vi "readTelemetryFPGAData.vi"(8 "error in (no error)":errorcluster, 10 "Parser":refnum<class "U8ArrayParserAutoIndexing.lvclass">, 11 "M1M3SAL in":refnum<class "M1M3SAL.lvclass">) -> (0 "error out":errorcluster, 2 "EventSummaryState":variant, 3 "M1M3SAL out":refnum<class "M1M3SAL.lvclass">)   [LabVIEW 2016, in "M1M3SupportCommunicator.lvlib" / "M1M3SAL.lvclass"]
uses:
  M1M3SAL.lvclass
  Common_RT_Utilities/U8ArrayParserAutoIndexing/U8ArrayParserAutoIndexing.lvclass
  DataTypes/Topics/TelemetryFPGAData.ctl
  DataTypes/Topics/Parts/Timestamp.ctl
  DataTypes/Topics/M1M3SupportTopics.lvlib
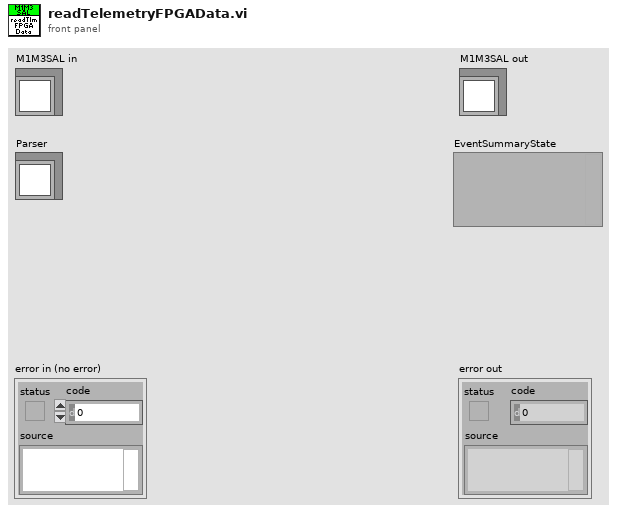
[diagram p1: front panel]
types:
  T1 = typedef "M1M3SupportTopics.lvlib/TelemetryFPGAData.ctl" = cluster{"Timestamp":T2, "ModbusSubnetATxInternalFIFOOverflow":bool, "ModbusSubnetAInvalidInstruction":bool, "ModbusSubnetAWaitForRxFrameTimeout":bool, "ModbusSubnetAStartBitError":bool, "ModbusSubnetAStopBitError":bool, "ModbusSubnetARxDataFIFOOverflow":bool, "ModbusSubnetATxByteCount":u32, "ModbusSubnetATxFrameCount":u32, "ModbusSubnetARxByteCount":u32, "ModbusSubnetARxFrameCount":u32, "ModbusSubnetBTxInternalFIFOOverflow":bool, "ModbusSubnetBInvalidInstruction":bool, "ModbusSubnetBWaitForRxFrameTimeout":bool, "ModbusSubnetBStartBitError":bool, "ModbusSubnetBStopBitError":bool, "ModbusSubnetBRxDataFIFOOverflow":bool, "ModbusSubnetBTxByteCount":u32, "ModbusSubnetBTxFrameCount":u32, "ModbusSubnetBRxByteCount":u32, "ModbusSubnetBRxFrameCount":u32, "ModbusSubnetCTxInternalFIFOOverflow":bool, "ModbusSubnetCInvalidInstruction":bool, "ModbusSubnetCWaitForRxFrameTimeout":bool, "ModbusSubnetCStartBitError":bool, "ModbusSubnetCStopBitError":bool, "ModbusSubnetCRxDataFIFOOverflow":bool, "ModbusSubnetCTxByteCount":u32, "ModbusSubnetCTxFrameCount":u32, "ModbusSubnetCRxByteCount":u32, "ModbusSubnetCRxFrameCount":u32, "ModbusSubnetDTxInternalFIFOOverflow":bool, "ModbusSubnetDInvalidInstruction":bool, "ModbusSubnetDWaitForRxFrameTimeout":bool, "ModbusSubnetDStartBitError":bool, "ModbusSubnetDStopBitError":bool, "ModbusSubnetDRxDataFIFOOverflow":bool, "ModbusSubnetDTxByteCount":u32, "ModbusSubnetDTxFrameCount":u32, "ModbusSubnetDRxByteCount":u32, "ModbusSubnetDRxFrameCount":u32, "ModbusSubnetETxInternalFIFOOverflow":bool, "ModbusSubnetEInvalidInstruction":bool, "ModbusSubnetEWaitForRxFrameTimeout":bool, "ModbusSubnetEStartBitError":bool, "ModbusSubnetEStopBitError":bool, "ModbusSubnetERxDataFIFOOverflow":bool, "ModbusSubnetETxByteCount":u32, "ModbusSubnetETxFrameCount":u32, "ModbusSubnetERxByteCount":u32, "ModbusSubnetERxFrameCount":u32, "FPGATimestamp":dbl}
  T2 = typedef "M1M3SupportTopics.lvlib/Timestamp.ctl" = dbl
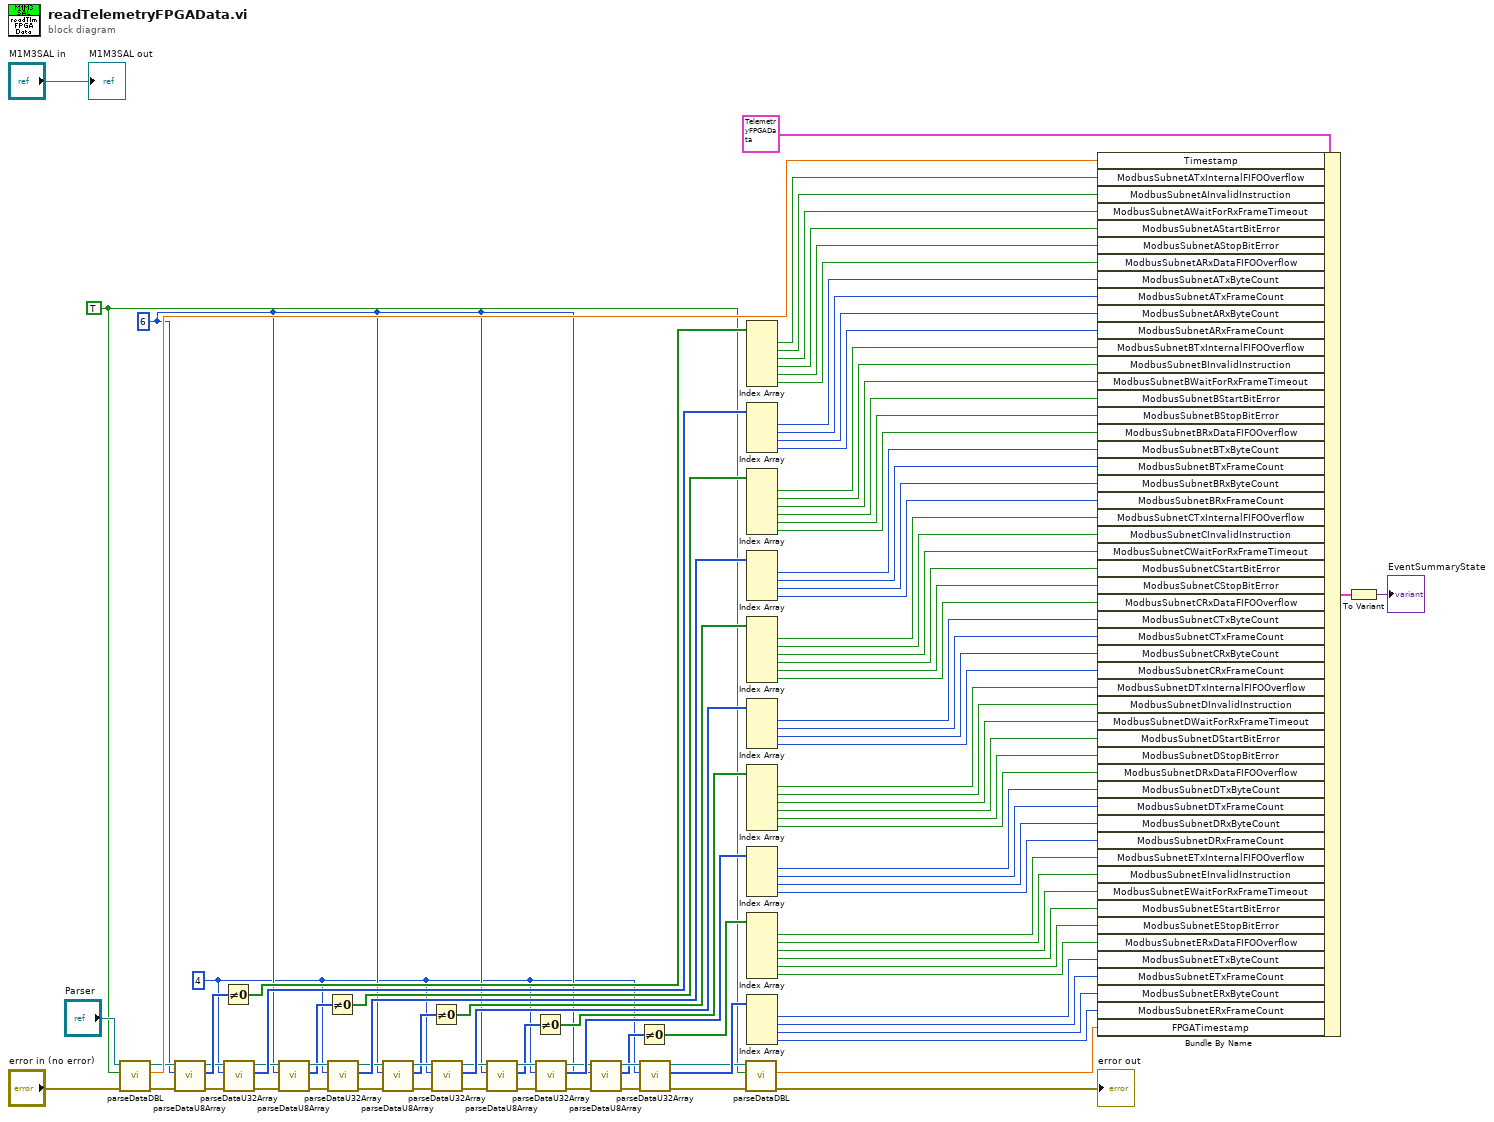
[diagram p0: block diagram]
diagram:
  w1 = TRUE ("OverrideSwapBytes")
  w2 = 4 ("Length")
  w3 = 6 ("Length")
  n1 = call "parseDataDBL.vi"("error in (no error)"="error in (no error)", "OverrideSwapBytes"=w1, "U8ArrayParserAutoIndexing in"="Parser") -> ("error out"=w76:errorcluster, "Data"=w94:dbl, "U8ArrayParserAutoIndexing out"=w79:refnum<class "U8ArrayParserAutoIndexing.lvclass">)  [unwired: 6 in]
  n2 = call "parseDataU8Array.vi"("U8ArrayParserAutoIndexing in"=w79, "Length"=w3, "error in (no error)"=w76) -> ("U8ArrayParserAutoIndexing out"=w78:refnum<class "U8ArrayParserAutoIndexing.lvclass">, "Data"=w92:u8[], "error out"=w75:errorcluster)  [unwired: 5 in]
  n3 = Not Equal To 0?(x=w92) -> (x != 0?=w91:bool[])
  n4 = call "parseDataU32Array.vi"("U8ArrayParserAutoIndexing in"=w78, "Length"=w2, "error in (no error)"=w75) -> ("U8ArrayParserAutoIndexing out"=w77:refnum<class "U8ArrayParserAutoIndexing.lvclass">, "Data"=w83:u32[], "error out"=w74:errorcluster)  [unwired: 5 in]
  n5 = call "parseDataU8Array.vi"("U8ArrayParserAutoIndexing in"=w77, "Length"=w3, "error in (no error)"=w74) -> ("U8ArrayParserAutoIndexing out"=w73:refnum<class "U8ArrayParserAutoIndexing.lvclass">, "Data"=w72:u8[], "error out"=w12:errorcluster)  [unwired: 5 in]
  n6 = Not Equal To 0?(x=w72) -> (x != 0?=w71:bool[])
  n7 = call "parseDataU32Array.vi"("U8ArrayParserAutoIndexing in"=w73, "Length"=w2, "error in (no error)"=w12) -> ("U8ArrayParserAutoIndexing out"=w69:refnum<class "U8ArrayParserAutoIndexing.lvclass">, "Data"=w70:u32[], "error out"=w11:errorcluster)  [unwired: 5 in]
  n8 = call "parseDataU8Array.vi"("U8ArrayParserAutoIndexing in"=w69, "Length"=w3, "error in (no error)"=w11) -> ("U8ArrayParserAutoIndexing out"=w68:refnum<class "U8ArrayParserAutoIndexing.lvclass">, "Data"=w67:u8[], "error out"=w10:errorcluster)  [unwired: 5 in]
  n9 = Not Equal To 0?(x=w67) -> (x != 0?=w66:bool[])
  n10 = call "parseDataU32Array.vi"("U8ArrayParserAutoIndexing in"=w68, "Length"=w2, "error in (no error)"=w10) -> ("U8ArrayParserAutoIndexing out"=w64:refnum<class "U8ArrayParserAutoIndexing.lvclass">, "Data"=w65:u32[], "error out"=w9:errorcluster)  [unwired: 5 in]
  n11 = call "parseDataU8Array.vi"("U8ArrayParserAutoIndexing in"=w64, "Length"=w3, "error in (no error)"=w9) -> ("U8ArrayParserAutoIndexing out"=w63:refnum<class "U8ArrayParserAutoIndexing.lvclass">, "Data"=w62:u8[], "error out"=w8:errorcluster)  [unwired: 5 in]
  n12 = Not Equal To 0?(x=w62) -> (x != 0?=w61:bool[])
  n13 = call "parseDataU32Array.vi"("U8ArrayParserAutoIndexing in"=w63, "Length"=w2, "error in (no error)"=w8) -> ("U8ArrayParserAutoIndexing out"=w59:refnum<class "U8ArrayParserAutoIndexing.lvclass">, "Data"=w60:u32[], "error out"=w7:errorcluster)  [unwired: 5 in]
  n14 = call "parseDataU8Array.vi"("U8ArrayParserAutoIndexing in"=w59, "Length"=w3, "error in (no error)"=w7) -> ("U8ArrayParserAutoIndexing out"=w58:refnum<class "U8ArrayParserAutoIndexing.lvclass">, "Data"=w57:u8[], "error out"=w6:errorcluster)  [unwired: 5 in]
  n15 = Not Equal To 0?(x=w57) -> (x != 0?=w56:bool[])
  n16 = call "parseDataU32Array.vi"("U8ArrayParserAutoIndexing in"=w58, "Length"=w2, "error in (no error)"=w6) -> ("U8ArrayParserAutoIndexing out"=w54:refnum<class "U8ArrayParserAutoIndexing.lvclass">, "Data"=w55:u32[], "error out"=w5:errorcluster)  [unwired: 5 in]
  n17 = call "parseDataDBL.vi"("error in (no error)"=w5, "OverrideSwapBytes"=w1, "U8ArrayParserAutoIndexing in"=w54) -> ("error out"=→"error out":errorcluster, "Data"=w53:dbl)  [unwired: 6 in, 1 out]
  n18 = Index Array(array=w91) -> (element #1=w90:bool, element #2=w89:bool, element #3=w88:bool, element #4=w87:bool, element #5=w86:bool, element #6=w85:bool)  [unwired: 6 in]
  n19 = Index Array(array=w83) -> (element #1=w84:u32, element #2=w82:u32, element #3=w81:u32, element #4=w80:u32)  [unwired: 4 in]
  n20 = Index Array(array=w71) -> (element #1=w52:bool, element #2=w51:bool, element #3=w50:bool, element #4=w49:bool, element #5=w48:bool, element #6=w47:bool)  [unwired: 6 in]
  n21 = Index Array(array=w70) -> (element #1=w46:u32, element #2=w45:u32, element #3=w44:u32, element #4=w43:u32)  [unwired: 4 in]
  n22 = Index Array(array=w66) -> (element #1=w42:bool, element #2=w41:bool, element #3=w40:bool, element #4=w39:bool, element #5=w38:bool, element #6=w37:bool)  [unwired: 6 in]
  n23 = Index Array(array=w65) -> (element #1=w36:u32, element #2=w35:u32, element #3=w34:u32, element #4=w33:u32)  [unwired: 4 in]
  n24 = Index Array(array=w61) -> (element #1=w32:bool, element #2=w31:bool, element #3=w30:bool, element #4=w29:bool, element #5=w28:bool, element #6=w27:bool)  [unwired: 6 in]
  n25 = Index Array(array=w60) -> (element #1=w26:u32, element #2=w25:u32, element #3=w24:u32, element #4=w23:u32)  [unwired: 4 in]
  n26 = Index Array(array=w56) -> (element #1=w22:bool, element #2=w21:bool, element #3=w20:bool, element #4=w19:bool, element #5=w18:bool, element #6=w17:bool)  [unwired: 6 in]
  n27 = Index Array(array=w55) -> (element #1=w16:u32, element #2=w15:u32, element #3=w14:u32, element #4=w13:u32)  [unwired: 4 in]
  n28 = Bundle By Name(cluster=T1 {"Timestamp"=0.0, "ModbusSubnetATxInternalFIFOOverflow"=FALSE, "ModbusSubnetAInvalidInstruction"=FALSE, "ModbusSubnetAWaitForRxFrameTimeout"=FALSE, "ModbusSubnetAStartBitError"=FALSE, "ModbusSubnetAStopBitError"=FALSE, "ModbusSubnetARxDataFIFOOverflow"=FALSE, "ModbusSubnetATxByteCount"=0, "ModbusSubnetATxFrameCount"=0, "ModbusSubnetARxByteCount"=0, "ModbusSubnetARxFrameCount"=0, "ModbusSubnetBTxInternalFIFOOverflow"=FALSE, "ModbusSubnetBInvalidInstruction"=FALSE, "ModbusSubnetBWaitForRxFrameTimeout"=FALSE, "ModbusSubnetBStartBitError"=FALSE, "ModbusSubnetBStopBitError"=FALSE, "ModbusSubnetBRxDataFIFOOverflow"=FALSE, "ModbusSubnetBTxByteCount"=0, "ModbusSubnetBTxFrameCount"=0, "ModbusSubnetBRxByteCount"=0, "ModbusSubnetBRxFrameCount"=0, "ModbusSubnetCTxInternalFIFOOverflow"=FALSE, "ModbusSubnetCInvalidInstruction"=FALSE, "ModbusSubnetCWaitForRxFrameTimeout"=FALSE, "ModbusSubnetCStartBitError"=FALSE, "ModbusSubnetCStopBitError"=FALSE, "ModbusSubnetCRxDataFIFOOverflow"=FALSE, "ModbusSubnetCTxByteCount"=0, "ModbusSubnetCTxFrameCount"=0, "ModbusSubnetCRxByteCount"=0, "ModbusSubnetCRxFrameCount"=0, "ModbusSubnetDTxInternalFIFOOverflow"=FALSE, "ModbusSubnetDInvalidInstruction"=FALSE, "ModbusSubnetDWaitForRxFrameTimeout"=FALSE, "ModbusSubnetDStartBitError"=FALSE, "ModbusSubnetDStopBitError"=FALSE, "ModbusSubnetDRxDataFIFOOverflow"=FALSE, "ModbusSubnetDTxByteCount"=0, "ModbusSubnetDTxFrameCount"=0, "ModbusSubnetDRxByteCount"=0, "ModbusSubnetDRxFrameCount"=0, "ModbusSubnetETxInternalFIFOOverflow"=FALSE, "ModbusSubnetEInvalidInstruction"=FALSE, "ModbusSubnetEWaitForRxFrameTimeout"=FALSE, "ModbusSubnetEStartBitError"=FALSE, "ModbusSubnetEStopBitError"=FALSE, "ModbusSubnetERxDataFIFOOverflow"=FALSE, "ModbusSubnetETxByteCount"=0, "ModbusSubnetETxFrameCount"=0, "ModbusSubnetERxByteCount"=0, "ModbusSubnetERxFrameCount"=0, "FPGATimestamp"=0.0} ("TelemetryFPGAData"), "Timestamp"=w94, "ModbusSubnetATxInternalFIFOOverflow"=w90, "ModbusSubnetAInvalidInstruction"=w89, "ModbusSubnetAWaitForRxFrameTimeout"=w88, "ModbusSubnetAStartBitError"=w87, "ModbusSubnetAStopBitError"=w86, "ModbusSubnetARxDataFIFOOverflow"=w85, "ModbusSubnetATxByteCount"=w84, "ModbusSubnetATxFrameCount"=w82, "ModbusSubnetARxByteCount"=w81, "ModbusSubnetARxFrameCount"=w80, "ModbusSubnetBTxInternalFIFOOverflow"=w52, "ModbusSubnetBInvalidInstruction"=w51, "ModbusSubnetBWaitForRxFrameTimeout"=w50, "ModbusSubnetBStartBitError"=w49, "ModbusSubnetBStopBitError"=w48, "ModbusSubnetBRxDataFIFOOverflow"=w47, "ModbusSubnetBTxByteCount"=w46, "ModbusSubnetBTxFrameCount"=w45, "ModbusSubnetBRxByteCount"=w44, "ModbusSubnetBRxFrameCount"=w43, "ModbusSubnetCTxInternalFIFOOverflow"=w42, "ModbusSubnetCInvalidInstruction"=w41, "ModbusSubnetCWaitForRxFrameTimeout"=w40, "ModbusSubnetCStartBitError"=w39, "ModbusSubnetCStopBitError"=w38, "ModbusSubnetCRxDataFIFOOverflow"=w37, "ModbusSubnetCTxByteCount"=w36, "ModbusSubnetCTxFrameCount"=w35, "ModbusSubnetCRxByteCount"=w34, "ModbusSubnetCRxFrameCount"=w33, "ModbusSubnetDTxInternalFIFOOverflow"=w32, "ModbusSubnetDInvalidInstruction"=w31, "ModbusSubnetDWaitForRxFrameTimeout"=w30, "ModbusSubnetDStartBitError"=w29, "ModbusSubnetDStopBitError"=w28, "ModbusSubnetDRxDataFIFOOverflow"=w27, "ModbusSubnetDTxByteCount"=w26, "ModbusSubnetDTxFrameCount"=w25, "ModbusSubnetDRxByteCount"=w24, "ModbusSubnetDRxFrameCount"=w23, "ModbusSubnetETxInternalFIFOOverflow"=w22, "ModbusSubnetEInvalidInstruction"=w21, "ModbusSubnetEWaitForRxFrameTimeout"=w20, "ModbusSubnetEStartBitError"=w19, "ModbusSubnetEStopBitError"=w18, "ModbusSubnetERxDataFIFOOverflow"=w17, "ModbusSubnetETxByteCount"=w16, "ModbusSubnetETxFrameCount"=w15, "ModbusSubnetERxByteCount"=w14, "ModbusSubnetERxFrameCount"=w13, "FPGATimestamp"=w53) -> (w98:T1)
  n29 = To Variant(anything=w98) -> (Variant=→"EventSummaryState":variant)
  "M1M3SAL out" <- "M1M3SAL in"
